vi "test_F9P_232-2.vi"() -> ()   [LabVIEW 2019]
panel:
  in  "cfg":T1={"Port"="COM5", "heading select"="NARROW_INT", "mode select"=["INS_RTKFIXED", "INS_RTKFLOAT"]}
  out "gps receive":string="$GNRMC,064134.00,A,3723.59859,N,12656.92614,E,0.021,,250720,,,A,V*12\r\n$GNVTG,,T,,M,0.021,N,0.039,K,A*34\r\n$GNGGA,064134.00,3723.59859,N,12656.92614,E,1,12,0.65,65.4,M,18.5,M,,*7E\r\n$GNGSA,A,3,17,19,06,05,02,12,09,,,,,,1.13,0.65,0.92,1*0F\r\n$GNGSA,A,3,85,70,71,72,,,,,,,,,1.13,0.65,0.92,2*00\r\n$GNGSA,A,3,36,19,11,04,09,12,,,,,,,1.13,0.65,0.92,3*0B\r\n$GNGSA,A,3,28,14,13,11,33,08,10,,,,,,1.13,0.65,0.92,4*0B\r\n$GPGSV,4,1,13,02,64,333,46,04,09,037,16,05,47,260,36,06,59,075,39,1*69\r\n$GPGSV,4,2,13,07,06,105,,09,39,058,39,12,18,264,15,13,07,191,,1*63\r\n$GPGSV,4,3,13,17,20,157,15,19,38,161,44,25,11,294,,29,06,323,,1*60\r\n$GPGSV,4,4,13,30,01,134,,1*52\r\n$GPGSV,4,1,13,02,64,333,,04,09,037,,05,47,260,36,06,59,075,37,6*65\r\n$GPGSV,4,2,13,07,06,105,,09,39,058,34,12,18,264,,13,07,191,,6*6D\r\n$GPGSV,4,3,13,17,20,157,,19,38,161,,25,11,294,,29,06,323,,6*63\r\n$GPGSV,4,4,13,30,01,134,,6*55\r\n$GLGSV,2,1,06,70,55,030,37,71,68,223,38,72,17,216,19,84,09,133,09,1*7E\r\n$GLGSV,2,2,06,85,64,109,38,86,50,337,,1*7E\r\n$GLGSV,2,1,06,70,55,030,,71,68,223,35,72,17,216,23,84,09,133,09,3*7C\r\n$GLGSV,2,2,06,85,64,109,33,86,50,337,,3*77\r\n$GAGSV,3,1,09,02,04,288,07,04,68,087,34,09,43,196,30,11,77,034,38,7*76\r\n$GAGSV,3,2,09,12,32,114,26,18,55,286,43,19,18,042,13,25,01,241,,7*7F\r\n$GAGSV,3,3,09,36,34,314,26,7*4A\r\n$GAGSV,3,1,09,02,04,288,,04,68,087,40,09,43,196,36,11,77,034,36,2*7F\r\n$GAGSV,3,2,09,12,32,114,16,18,55,286,46,19,18,042,,25,01,241,,2*7E\r\n$GAGSV,3,3,09,36,34,314,25,2*4C\r\n$GBGSV,4,1,13,04,35,133,,05,09,257,,06,27,182,,07,09,201,,1*7B\r\n$GBGSV,4,2,13,08,65,355,42,09,07,194,,10,16,222,,11,38,142,24,1*70\r\n$GBGSV,4,3,13,13,50,314,28,14,77,038,43,28,58,310,41,33,72,237,40,1*76\r\n$GBGSV,4,4,13,34,13,141,,1*45\r\n$GBGSV,4,1,13,04,35,133,,05,09,257,,06,27,182,,07,09,201,,3*79\r\n$GBGSV,4,2,13,08,65,355,43,09,07,194,,10,16,222,17,11,38,142,22,3*73\r\n$GBGSV,4,3,13,13,50,314,32,14,77,038,42,28,58,310,,33,72,237,,3*7F\r\n$GBGSV,4,4,13,34,13,141,,3*47\r\n$GNGLL,3723.59859,N,12656.92614,E,064134.00,A,A*70\r\n$GNRMC,064135.00,A,3723.59865,N,12656.92610,E,0.011,,250720,,,A,V*1B\r\n$GNVTG,,T,,M,0.011,N,0.020,K,A*3F\r\n$GNGGA,064135.00,3723.59865,N,12656.92610,E,1,12,0.65,65.2,M,18.5,M,,*72\r\n$GNGSA,A,3,17,19,06,05,02,12,09,,,,,,1.13,0.65,0.92,1*0F\r\n$GNGSA,A,3,85,70,71,72,,,,,,,,,1.13,0.65,0.92,2*00\r\n$GNGSA,A,3,36,19,11,04,09,12,,,,,,,1.13,0.65,0.92,3*0B\r\n$GNGSA,A,3,28,14,13,11,33,08,10,,,,,,1.13,0.65,0.92,4*0B\r\n$GPGSV,4,1,13,02,64,333,45,04,09,037,16,05,47,260,37,06,59,075,39,1*6B\r\n$GPGSV,4,2,13,07,06,105,,09,39,058,39,12,18,264,14,13,07,191,,1*62\r\n$GPGSV,4,3,13,17,20,157,16,19,38,161,44,25,11,294,,29,06,323,17,1*65\r\n$GPGSV,4,4,13,30,01,134,,1*52\r\n$GPGSV,4,1,13,02,64,333,,04,09,037,,05,47,260,35,06,59,075,37,6*66\r\n$GPGSV,4,2,13,07,06,105,,09,39,058,34,12,18,264,,13,07,191,,6*6D\r\n$GPGSV,4,3,13,17,20,157,,19,38,161,,25,11,294,,29,06,323,,6*63\r\n$GPGSV,4,4,13,30,01,134,,6*55\r\n$GLGSV,2,1,06,70,55,030,37,71,68,223,40,72,17,216,18,84,09,133,12,1*7A\r\n$GLGSV,2,2,06,85,64,109,38,86,50,337,,1*7E\r\n$GLGSV,2,1,06,70,55,030,,71,68,223,37,72,17,216,23,84,09,133,08,3*7F\r\n$GLGSV,2,2,06,85,64,109,33,86,50,337,,3*77\r\n$GAGSV,3,1,09,02,04,288,11,04,68,087,34,09,43,196,30,11,77,034,38,7*71\r\n$GAGSV,3,2,09,12,32,114,26,18,55,286,43,19,18,042,12,25,01,241,,7*7E\r\n$GAGSV,3,3,09,36,34,314,26,7*4A\r\n$GAGSV,3,1,09,02,04,288,,04,68,087,40,09,43,196,36,11,77,034,36,2*7F\r\n$GAGSV,3,2,09,12,32,114,16,18,55,286,47,19,18,042,,25,01,241,,2*7F\r\n$GAGSV,3,3,09,36,34,314,25,2*4C\r\n$GBGSV,4,1,13,04,35,133,,05,09,257,,06,27,182,,07,09,201,,1*7B\r\n$GBGSV,4,2,13,08,65,355,41,09,07,194,,10,16,222,,11,38,142,23,1*74\r\n$GBGSV,4,3,13,13,50,314,28,14,77,038,43,28,58,310,41,33,72,237,40,1*76\r\n$GBGSV,4,4,13,34,13,141,,1*45\r\n$GBGSV,4,1,13,04,35,133,,05,09,257,,06,27,182,,07,09,201,,3*79\r\n$GBGSV,4,2,13,08,65,355,43,09,07,194,,10,16,222,18,11,38,142,21,3*7F\r\n$GBGSV,4,3,13,13,50,314,31,14,77,038,41,28,58,310,,33,72,237,,3*7F\r\n$GBGSV,4,4,13,34,13,141,,3*47\r\n$GNGLL,3723.59865,N,12656.92610,E,064135.00,A,A*7A\r\n$GNRMC,064136.00,A,3723.59874,N,12656.92610,E,0.025,,250720,,,A,V*1F\r\n$GNVTG,,T,,M,0.025,N,0.046,K,A*38\r\n$GNGGA,064136.00,3723.59874,N,12656.92610,E,1,12,0.65,65.2,M,18.5,M,,*71\r\n$GNGSA,A,3,17,19,06,05,02,12,09,,,,,,1.13,0.65,0.92,1*0F\r\n$GNGSA,A,3,85,70,71,72,,,,,,,,,1.13,0.65,0.92,2*00\r\n$GNGSA,A,3,36,19,11,04,09,12,,,,,,,1.13,0.65,0.92,3*0B\r\n$GNGSA,A,3,28,14,13,11,33,08,10,,,,,,1.13,0.65,0.92,4*0B\r\n$GPGSV,4,1,13,02,64,333,43,04,09,037,15,05,47,260,30,06,59,075,36,1*66\r\n$GPGSV,4,2,13,07,06,105,,09,39,058,39,12,18,264,15,13,07,191,,1*63\r\n$GPGSV,4,3,13,17,20,157,14,19,38,161,41,25,11,294,,29,06,323,18,1*6D\r\n$GPGSV,4,4,13,30,01,134,,1*52\r\n$GPGSV,4,1,13,02,64,333,,04,09,037,,05,47,260,35,06,59,075,37,6*66\r\n$GPGSV,4,2,13,07,06,105,,09,39,058,34,12,18,264,,13,07,191,,6*6D\r\n$GPGSV,4,3,13,17,20,157,,19,38,161,,25,11,294,,29,06,323,,6*63\r\n$GPGSV,4,4,13,30,01,134,,6*55\r\n$GLGSV,2,1,06,70,55,030,35,71,68,223,38,72,17,216,17,84,09,133,09,1*72\r\n$GLGSV,2,2,06,85,64,109,34,86,50,337,,1*72\r\n$GLGSV,2,1,06,70,55,030,,71,68,223,37,72,17,216,24,84,09,133,11,3*70\r\n$GLGSV,2,2,06,85,64,109,35,86,50,337,,3*71\r\n$GAGSV,3,1,09,02,04,288,07,04,68,087,33,09,43,196,30,11,77,034,36,7*7F\r\n$GAGSV,3,2,09,12,32,114,26,18,55,286,41,19,18,042,13,25,01,241,,7*7D\r\n$GAGSV,3,3,09,36,34,314,27,7*4B\r\n$GAGSV,3,1,09,02,04,288,,04,68,087,40,09,43,196,37,11,77,034,36,2*7E\r\n$GAGSV,3,2,09,12,32,114,17,18,55,286,46,19,18,042,,25,01,241,,2*7F\r\n$GAGSV,3,3,09,36,34,314,25,2*4C\r\n$GBGSV,4,1,13,04,35,133,,05,09,257,,06,27,182,,07,09,201,,1*7B\r\n$GBGSV,4,2,13,08,65,355,40,09,07,194,,10,16,222,,11,38,142,22,1*74\r\n$GBGSV,4,3,13,13,50,314,28,14,77,038,41,28,58,310,42,33,72,237,39,1*79\r\n$GBGSV,4,4,13,34,13,141,,1*45\r\n$GBGSV,4,1,13,04,35,133,,05,09,257,,06,27,182,,07,09,201,,3*79\r\n$GBGSV,4,2,13,08,65,355,42,09,07,194,,10,16,222,19,11,38,142,19,3*74\r\n$GBGSV,4,3,13,13,50,314,31,14,77,038,41,28,58,310,,33,72,237,,3*7F\r\n$GBGSV,4,4,13,34,13,141,,3*47\r\n$GNGLL,3723.59874,N,12656.92610,E,064136.00,A,A*79\r\n$GNRMC,064137.00,A,3723.59883,N,12656.92607,E,0.046,,250720,,,A,V*15\r\n$GNVTG,,T,,M,0.046,N,0.085,K,A*32\r\n$GNGGA,064137.00,3723.59883,N,12656.92607,E,1,12,0.65,65.5,M,18.5,M,,*79\r\n$GNGSA,A,3,17,19,06,05,02,12,09,,,,,,1.13,0.65,0.92,1*0F\r\n$GNGSA,A,3,85,70,71,72,,,,,,,,,1.13,0.65,0.92,2*00\r\n$GNGSA,A,3,36,19,11,04,09,12,,,,,,,1.13,0.65,0.92,3*0B\r\n$GNGSA,A,3,28,14,13,11,33,08,10,,,,,,1.13,0.65,0.92,4*0B\r\n$GPGSV,4,1,13,02,64,333,46,04,09,037,12,05,47,260,32,06,59,075,43,1*64\r\n$GPGSV,4,2,13,07,06,105,,09,39,058,32,12,18,264,17,13,07,191,,1*6A\r\n$GPGSV,4,3,13,17,20,157,13,19,38,161,43,25,11,294,,29,06,323,17,1*67\r\n$GPGSV,4,4,13,30,01,134,,1*52\r\n$GPGSV,4,1,13,02,64,333,,04,09,037,,05,47,260,35,06,59,075,37,6*66\r\n$GPGSV,4,2,13,07,06,105,,09,39,058,35,12,18,264,,13,07,191,,6*6C\r\n$GPGSV,4,3,13,17,20,157,,19,38,161,,25,11,294,,29,06,323,,6*63\r\n$GPGSV,4,4,13,30,01,134,,6*55\r\n$GLGSV,2,1,06,70,55,030,36,71,68,223,42,72,17,216,18,84,09,133,09,1*73\r\n$GLGSV,2,2,06,85,64,109,37,86,50,337,,1*71\r\n$GLGSV,2,1,06,70,55,030,,71,68,223,36,72,17,216,24,84,09,133,10,3*70\r\n$GLGSV,2,2,06,85,64,109,33,86,50,337,,3*77\r\n$GAGSV,3,1,09,02,04,288,10,04,68,087,37,09,43,196,30,11,77,034,38,7*73\r\n$GAGSV,3,2,09,12,32,114,26,18,55,286,45,19,18,042,14,25,01,241,,7*7E\r\n$GAGSV,3,3,09,36,34,314,28,7*44\r\n$GAGSV,3,1,09,02,04,288,,04,68,087,40,09,43,196,37,11,77,034,37,2*7F\r\n$GAGSV,3,2,09,12,32,114,16,18,55,286,47,19,18,042,,25,01,241,,2*7F\r\n$GAGSV,3,3,09,36,34,314,25,2*4C\r\n$GBGSV,4,1,13,04,35,133,,05,09,257,,06,27,182,,07,09,201,,1*7B\r\n$GBGSV,4,2,13,08,65,355,40,09,07,194,,10,16,222,,11,38,142,21,1*77\r\n$GBGSV,4,3,13,13,50,314,29,14,77,038,43,28,58,310,41,33,72,237,40,1*77\r\n$GBGSV,4,4,13,34,13,141,,1*45\r\n$GBGSV,4,1,13,04,35,133,,05,09,257,,06,27,182,,07,09,201,,3*79\r\n$GBGSV,4,2,13,08,65,355,44,09,07,194,,10,16,222,18,11,38,142,18,3*72\r\n$GBGSV,4,3,13,13,50,314,32,14,77,038,42,28,58,310,,33,72,237,,3*7F\r\n$GBGSV,4,4,13,34,13,141,,3*47\r\n$GNGLL,3723.59883,N,12656.92607,E,064137.00,A,A*76\r\n$GNRMC,064138.00,A,3723.59888,N,12656.92600,E,0.018,,250720,,,A,V*1D\r\n$GNVTG,,T,,M,0.018,N,0.033,K,A*34\r\n$GNGGA,064138.00,3723.59888,N,12656.92600,E,1,12,0.70,65.3,M,18.5,M,,*78\r\n$GNGSA,A,3,17,19,06,05,02,09,,,,,,,1.20,0.70,0.98,1*02\r\n$GNGSA,A,3,85,70,71,72,,,,,,,,,1.20,0.70,0.98,2*0E\r\n$GNGSA,A,3,36,19,11,04,09,12,,,,,,,1.20,0.70,0.98,3*05\r\n$GNGSA,A,3,28,14,13,11,33,08,10,,,,,,1.20,0.70,0.98,4*05\r\n$GPGSV,4,1,13,02,64,333,45,04,09,037,,05,47,260,38,06,59,075,43,1*6E\r\n$GPGSV,4,2,13,07,06,105,,09,39,058,32,12,18,264,,13,07,191,,1*6C\r\n$GPGSV,4,3,13,17,20,157,15,19,38,161,42,25,11,294,,29,06,323,18,1*6F\r\n$GPGSV,4,4,13,30,01,134,,1*52\r\n$GPGSV,4,1,13,02,64,333,,04,09,037,,05,47,260,36,06,59,075,35,6*67\r\n$GPGSV,4,2,13,07,06,105,,09,39,058,34,12,18,264,,13,07,191,,6*6D\r\n$GPGSV,4,3,13,17,20,157,,19,38,161,,25,11,294,,29,06,323,,6*63\r\n$GPGSV,4,4,13,30,01,134,,6*55\r\n$GLGSV,2,1,06,70,55,030,40,71,68,223,42,72,17,216,19,84,09,133,14,1*7F\r\n$GLGSV,2,2,06,85,63,111,40,86,50,337,,1*7F\r\n$GLGSV,2,1,06,70,55,030,,71,68,223,36,72,17,216,25,84,09,133,09,3*79\r\n$GLGSV,2,2,06,85,63,111,28,86,50,337,,3*73\r\n$GAGSV,3,1,09,02,04,288,09,04,68,087,36,09,43,196,33,11,77,034,38,7*79\r\n$GAGSV,3,2,09,12,32,114,23,18,55,286,45,19,18,042,12,25,01,241,,7*7D\r\n$GAGSV,3,3,09,36,34,314,26,7*4A\r\n$GAGSV,3,1,09,02,04,288,,04,68,087,41,09,43,196,36,11,77,034,37,2*7F\r\n$GAGSV,3,2,09,12,32,114,15,18,55,286,48,19,18,042,,25,01,241,,2*73\r\n$GAGSV,3,3,09,36,34,314,24,2*4D\r\n$GBGSV,4,1,13,04,35,133,,05,09,257,,06,27,182,,07,09,201,,1*7B\r\n$GBGSV,4,2,13,08,65,355,40,09,07,194,,10,16,222,,11,38,142,21,1*77\r\n$GBGSV,4,3,13,13,50,314,32,14,77,038,43,28,58,310,43,33,72,237,41,1*7E\r\n$GBGSV,4,4,13,34,13,141,,1*45\r\n$GBGSV,4,1,13,04,35,133,,05,09,257,,06,27,182,,07,09,201,,3*79\r\n$GBGSV,4,2,13,08,65,355,44,09,07,194,,10,16,222,18,11,38,142,17,3*7D\r\n$GBGSV,4,3,13,13,50,314,31,14,77,038,43,28,58,310,,33,72,237,,3*7D\r\n$GBGSV,4,4,13,34,13,141,,3*47\r\n$GNGLL,3723.59888,N,12656.92600,E,064138.00,A,A*75\r\n$GNRMC,064139.00,A,3723.59894,N,12656.92597,E,0.040,,250720,,,A,V*11\r\n$GNVTG,,T,,M,0.040,N,0.073,K,A*3D\r\n$GNGGA,064139.00,3723.59894,N,12656.92597,E,1,12,0.76,65.2,M,18.5,M,,*7E\r\n$GNGSA,A,3,17,19,06,05,02,09,,,,,,,1.26,0.76,1.01,1*03\r\n$GNGSA,A,3,85,70,71,72,,,,,,,,,1.26,0.76,1.01,2*0F\r\n$GNGSA,A,3,36,19,11,04,09,12,,,,,,,1.26,0.76,1.01,3*04\r\n$GNGSA,A,3,28,14,13,11,33,08,10,,,,,,1.26,0.76,1.01,4*04\r\n$GPGSV,4,1,13,02,64,333,44,04,09,037,,05,47,260,37,06,59,075,40,1*63\r\n$GPGSV,4,2,13,07,06,105,,09,39,058,35,12,18,264,,13,07,191,,1*6B\r\n$GPGSV,4,3,13,17,20,157,14,19,38,161,42,25,11,294,,29,06,323,18,1*6E\r\n$GPGSV,4,4,13,30,01,134,,1*52\r\n$GPGSV,4,1,13,02,64,333,,04,09,037,,05,47,260,36,06,59,075,36,6*64\r\n$GPGSV,4,2,13,07,06,105,,09,39,058,37,12,18,264,,13,07,191,,6*6E\r\n$GPGSV,4,3,13,17,20,157,,19,38,161,,25,11,294,,29,06,323,,6*63\r\n$GPGSV,4,4,13,30,01,134,,6*55\r\n$GLGSV,2,1,06,70,55,030,39,71,68,223,43,72,17,216,21,84,09,133,11,1*7E\r\n$GLGSV,2,2,06,85,63,111,41,86,51,337,,1*7F\r\n$GLGSV,2,1,06,70,55,030,,71,68,223,35,72,17,216,24,84,09,133,08,3*7A\r\n$GLGSV,2,2,06,85,63,111,27,86,51,337,,3*7D\r\n$GAGSV,3,1,09,02,04,288,08,04,68,087,38,09,43,196,27,11,77,034,38,7*73\r\n$GAGSV,3,2,09,12,32,114,25,18,55,286,45,19,18,042,13,25,01,241,,7*7A\r\n$GAGSV,3,3,09,36,34,314,25,7*49\r\n$GAGSV,3,1,09,02,04,288,,04,68,087,41,09,43,196,37,11,77,034,37,2*7E\r\n$GAGSV,3,2,09,12,32,114,13,18,55,286,47,19,18,042,,25,01,241,,2*7A\r\n$GAGSV,3,3,09,36,34,314,24,2*4D\r\n$GBGSV,4,1,13,04,35,133,,05,09,257,,06,27,182,,07,09,201,,1*7B\r\n$GBGSV,4,2,13,08,65,355,39,09,07,194,,10,16,222,,11,38,142,20,1*78\r\n$GBGSV,4,3,13,13,50,314,33,14,77,038,42,28,58,310,40,33,72,237,41,1*7D\r\n$GBGSV,4,4,13,34,13,141,,1*45\r\n$GBGSV,4,1,13,04,35,133,,05,09,257,,06,27,182,,07,09,201,,3*79\r\n$GBGSV,4,2,13,08,65,355,44,09,07,194,,10,16,222,17,11,38,142,17,3*72\r\n$GBGSV,4,3,13,13,50,314,30,14,77,038,42,28,58,310,,33,72,237,,3*7D\r\n$GBGSV,4,4,13,34,13,141,,3*47\r\n$GNGLL,3723.59894,N,12656.92597,E,064139.00,A,A*74\r\n$GNRMC,064140.00,A,3723.59897,N,12656.92595,E,0.024,,250720,,,A,V*1C\r\n$GNVTG,,T,,M,0.024,N,0.044,K,A*3B\r\n$GNGGA,064140.00,3723.59897,N,12656.92595,E,1,12,0.76,64.8,M,18.5,M,,*7A\r\n$GNGSA,A,3,19,06,05,02,09,,,,,,,,1.26,0.76,1.01,1*05\r\n$GNGSA,A,3,85,70,71,72,,,,,,,,,1.26,0.76,1.01,2*0F\r\n$GNGSA,A,3,36,19,11,04,09,12,,,,,,,1.26,0.76,1.01,3*04\r\n$GNGSA,A,3,28,14,13,11,33,08,10,,,,,,1.26,0.76,1.01,4*04\r\n$GPGSV,4,1,13,02,64,333,47,04,09,037,,05,47,260,36,06,59,075,39,1*6F\r\n$GPGSV,4,2,13,07,06,105,,09,39,058,35,12,18,264,,13,07,191,,1*6B\r\n$GPGSV,4,3,13,17,20,157,,19,38,161,43,25,11,294,,29,06,323,18,1*6A\r\n$GPGSV,4,4,13,30,01,134,,1*52\r\n$GPGSV,4,1,13,02,64,333,,04,09,037,,05,47,260,36,06,59,075,34,6*66\r\n$GPGSV,4,2,13,07,06,105,,09,39,058,37,12,18,264,,13,07,191,,6*6E\r\n$GPGSV,4,3,13,17,20,157,,19,38,161,,25,11,294,,29,06,323,,6*63\r\n$GPGSV,4,4,13,30,01,134,,6*55\r\n$GLGSV,2,1,06,70,55,030,39,71,68,223,43,72,17,216,22,84,09,133,13,1*7F\r\n$GLGSV,2,2,06,85,63,111,42,86,51,337,,1*7C\r\n$GLGSV,2,1,06,70,55,030,,71,68,223,37,72,17,216,23,84,09,133,08,3*7F\r\n$GLGSV,2,2,06,85,63,111,28,86,51,337,,3*72\r\n$GAGSV,3,1,09,02,04,288,08,04,68,087,39,09,43,196,31,11,77,034,38,7*75\r\n$GAGSV,3,2,09,12,32,114,26,18,55,286,45,19,18,042,11,25,01,241,,7*7B\r\n$GAGSV,3,3,09,36,34,314,25,7*49\r\n$GAGSV,3,1,09,02,04,288,,04,68,087,38,09,43,196,37,11,77,034,37,2*70\r\n$GAGSV,3,2,09,12,32,114,12,18,55,286,47,19,18,042,,25,01,241,,2*7B\r\n$GAGSV,3,3,09,36,34,314,23,2*4A\r\n$GBGSV,4,1,13,04,35,133,,05,09,257,,06,27,182,,07,09,201,,1*7B\r\n$GBGSV,4,2,13,08,65,355,41,09,07,194,,10,16,222,,11,38,142,22,1*75\r\n$GBGSV,4,3,13,13,50,314,33,14,77,038,43,28,58,310,41,33,72,237,43,1*7F\r\n$GBGSV,4,4,13,34,13,141,,1*45\r\n$GBGSV,4,1,13,04,35,133,,05,09,257,,06,27,182,,07,09,201,,3*79\r\n$GBGSV,4,2,13,08,65,355,44,09,07,194,,10,16,222,16,11,38,142,17,3*73\r\n$GBGSV,4,3,13,13,50,314,31,14,77,038,41,28,58,310,,33,72,237,,3*7F\r\n$GBGSV,4,4,13,34,13,141,,3*47\r\n$GNGLL,3723.59897,N,12656.92595,E,064140.00,A,A*7B\r\n$GNRMC,064141.00,A,3723.59895,N,12656.92586,E,0.013,,250720,,,A,V*19\r\n$GNVTG,,T,,M,0.013,N,0.024,K,A*39\r\n$GNGGA,064141.00,3723.59895,N,12656.92586,E,1,12,0.76,64.6,M,18.5,M,,*75\r\n$GNGSA,A,3,19,06,05,02,09,,,,,,,,1.26,0.76,1.01,1*05\r\n$GNGSA,A,3,85,70,71,72,,,,,,,,,1.26,0.76,1.01,2*0F\r\n$GNGSA,A,3,36,19,11,04,09,12,,,,,,,1.26,0.76,1.01,3*04\r\n$GNGSA,A,3,28,14,13,11,33,08,10,,,,,,1.26,0.76,1.01,4*04\r\n$GPGSV,4,1,13,02,64,333,45,04,09,037,,05,47,260,39,06,59,075,42,1*6E\r\n$GPGSV,4,2,13,07,06,105,,09,39,058,,12,18,264,,13,07,191,,1*6D\r\n$GPGSV,4,3,13,17,20,157,18,19,38,161,42,25,11,294,,29,06,323,18,1*62\r\n$GPGSV,4,4,13,30,01,134,,1*52\r\n$GPGSV,4,1,13,02,64,333,,04,09,037,,05,47,260,36,06,59,075,34,6*66\r\n$GPGSV,4,2,13,07,06,105,,09,39,058,34,12,18,264,,13,07,191,,6*6D\r\n$GPGSV,4,3,13,17,20,157,,19,38,161,,25,11,294,,29,06,323,,6*63\r\n$GPGSV,4,4,13,30,01,134,,6*55\r\n$GLGSV,2,1,06,70,55,030,36,71,68,223,44,72,17,216,21,84,09,133,11,1*76\r\n$GLGSV,2,2,06,85,63,111,37,86,51,337,,1*7E\r\n$GLGSV,2,1,06,70,55,030,,71,68,223,37,72,17,216,23,84,09,133,10,3*76\r\n$GLGSV,2,2,06,85,63,111,33,86,51,337,,3*78\r\n$GAGSV,3,1,09,02,04,288,11,04,68,087,36,09,44,196,31,11,77,034,40,7*7A\r\n$GAGSV,3,2,09,12,32,114,26,18,55,286,46,19,18,042,09,25,01,241,,7*71\r\n$GAGSV,3,3,09,36,34,314,25,7*49\r\n$GAGSV,3,1,09,02,04,288,,04,68,087,40,09,44,196,37,11,77,034,36,2*79\r\n$GAGSV,3,2,09,12,32,114,11,18,55,286,47,19,18,042,,25,01,241,,2*78\r\n$GAGSV,3,3,09,36,34,314,22,2*4B\r\n$GBGSV,4,1,13,04,35,133,,05,09,257,,06,27,182,,07,09,201,,1*7B\r\n$GBGSV,4,2,13,08,65,355,41,09,07,194,,10,16,222,,11,38,142,22,1*75\r\n$GBGSV,4,3,13,13,50,314,30,14,77,038,43,28,58,310,42,33,72,237,42,1*7E\r\n$GBGSV,4,4,13,34,13,141,,1*45\r\n$GBGSV,4,1,13,04,35,133,,05,09,257,,06,27,182,,07,09,201,,3*79\r\n$GBGSV,4,2,13,08,65,355,44,09,07,194,,10,16,222,16,11,38,142,19,3*7D\r\n$GBGSV,4,3,13,13,50,314,31,14,77,038,41,28,58,310,,33,72,237,,3*7F\r\n$GBGSV,4,4,13,34,13,141,,3*47\r\n$GNGLL,3723.59895,N,12656.92586,E,064141.00,A,A*7A\r\n$GNRMC,064142.00,A,3723.59893,N,12656.92582,E,0.128,,250720,,,A,V*11\r\n$GNVTG,,T,,M,0.128,N,0.238,K,A*3F\r\n$GNGGA,064142.00,3723.59893,N,12656.92582,E,1,12,0.76,64.4,M,18.5,M,,*76\r\n$GNGSA,A,3,19,06,05,02,09,,,,,,,,1.26,0.76,1.01,1*05\r\n$GNGSA,A,3,85,70,71,72,,,,,,,,,1.26,0.76,1.01,2*0F\r\n$GNGSA,A,3,36,19,11,04,09,12,,,,,,,1.26,0.76,1.01,3*04\r\n$GNGSA,A,3,28,14,13,11,33,08,10,,,,,,1.26,0.76,1.01,4*04\r\n$GPGSV,4,1,13,02,64,333,46,04,09,037,,05,47,260,39,06,59,075,45,1*6A\r\n$GPGSV,4,2,13,07,06,105,,09,39,058,37,12,18,264,19,13,07,191,,1*61\r\n$GPGSV,4,3,13,17,20,157,21,19,38,161,42,25,11,294,,29,06,323,17,1*67\r\n$GPGSV,4,4,13,30,01,134,,1*52\r\n$GPGSV,4,1,13,02,64,333,,04,09,037,,05,47,260,35,06,59,075,36,6*67\r\n$GPGSV,4,2,13,07,06,105,,09,39,058,34,12,18,264,,13,07,191,,6*6D\r\n$GPGSV,4,3,13,17,20,157,,19,38,161,,25,11,294,,29,06,323,,6*63\r\n$GPGSV,4,4,13,30,01,134,,6*55\r\n$GLGSV,2,1,06,70,55,030,34,71,68,223,37,72,17,216,21,84,09,133,10,1*71\r\n$GLGSV,2,2,06,85,63,111,39,86,51,337,,1*70\r\n$GLGSV,2,1,06,70,55,030,,71,68,223,33,72,17,216,23,84,09,133,08,3*7B\r\n$GLGSV,2,2,06,85,63,111,36,86,51,337,,3*7D\r\n$GAGSV,3,1,09,02,04,288,08,04,68,087,33,09,44,196,27,11,77,034,39,7*7E\r\n$GAGSV,3,2,09,12,32,114,25,18,55,286,48,19,18,042,16,25,01,241,,7*72\r\n$GAGSV,3,3,09,36,34,314,24,7*48\r\n$GAGSV,3,1,09,02,04,288,,04,68,087,40,09,44,196,37,11,77,034,36,2*79\r\n$GAGSV,3,2,09,12,32,114,12,18,55,286,45,19,18,042,,25,01,241,,2*79\r\n$GAGSV,3,3,09,36,34,314,22,2*4B\r\n$GBGSV,4,1,13,04,35,133,,05,09,257,,06,27,182,,07,09,201,,1*7B\r\n$GBGSV,4,2,13,08,65,355,42,09,07,194,,10,16,222,,11,38,142,25,1*71\r\n$GBGSV,4,3,13,13,50,314,33,14,77,038,42,28,58,310,41,33,72,237,37,1*7D\r\n$GBGSV,4,4,13,34,13,141,,1*45\r\n$GBGSV,4,1,13,04,35,133,,05,09,257,,06,27,182,,07,09,201,,3*79\r\n$GBGSV,4,2,13,08,65,355,42,09,07,194,,10,16,222,16,11,38,142,20,3*71\r\n$GBGSV,4,3,13,13,50,314,30,14,77,038,41,28,58,310,,33,72,237,,3*7E\r\n$GBGSV,4,4,13,34,13,141,,3*47\r\n$GNGLL,3723.59893,N,12656.92582,E,064142.00,A,A*7B\r\n$GNRMC,064143.00,A,3723.59889,N,12656.92573,E,0.182,,250720,,,A,V*15\r\n$GNVTG,,T,,M,0.182,N,0.338,K,A*3E\r\n$GNGGA,064143.00,3723.59889,N,12656.92573,E,1,12,0.68,64.4,M,18.5,M,,*7D\r\n$GNGSA,A,3,17,19,06,05,02,09,,,,,,,1.17,0.68,0.95,1*02\r\n$GNGSA,A,3,85,70,71,72,,,,,,,,,1.17,0.68,0.95,2*0E\r\n$GNGSA,A,3,36,19,11,04,09,12,,,,,,,1.17,0.68,0.95,3*05\r\n$GNGSA,A,3,28,14,13,11,33,08,10,,,,,,1.17,0.68,0.95,4*05\r\n$GPGSV,4,1,13,02,64,333,44,04,09,037,,05,47,260,40,06,59,075,36,1*62\r\n$GPGSV,4,2,13,07,06,105,,09,39,058,33,12,18,264,19,13,07,191,,1*65\r\n$GPGSV,4,3,13,17,20,157,23,19,38,161,39,25,11,294,,29,06,323,16,1*68\r\n$GPGSV,4,4,13,30,01,134,,1*52\r\n$GPGSV,4,1,13,02,64,333,,04,09,037,,05,47,260,34,06,59,075,34,6*64\r\n$GPGSV,4,2,13,07,06,105,,09,39,058,33,12,18,264,,13,07,191,,6*6A\r\n$GPGSV,4,3,13,17,20,157,,19,38,161,,25,11,294,,29,06,323,,6*63\r\n$GPGSV,4,4,13,30,01,134,,6*55\r\n$GLGSV,2,1,06,70,55,030,33,71,68,223,25,72,17,216,22,84,09,133,10,1*76\r\n$GLGSV,2,2,06,85,63,111,30,86,51,337,,1*79\r\n$GLGSV,2,1,06,70,55,030,,71,68,223,35,72,17,216,24,84,09,133,11,3*72\r\n$GLGSV,2,2,06,85,63,111,33,86,51,337,,3*78\r\n$GAGSV,3,1,09,02,04,288,07,04,68,087,38,09,44,196,27,11,77,034,38,7*7B\r\n$GAGSV,3,2,09,12,32,114,23,18,55,286,44,19,18,042,14,25,01,241,,7*7A\r\n$GAGSV,3,3,09,36,34,314,25,7*49\r\n$GAGSV,3,1,09,02,04,288,,04,68,087,37,09,44,196,35,11,77,034,30,2*7D\r\n$GAGSV,3,2,09,12,32,114,13,18,55,286,45,19,18,042,,25,01,241,,2*78\r\n$GAGSV,3,3,09,36,34,314,23,2*4A\r\n$GBGSV,4,1,13,04,35,133,,05,09,257,,06,27,182,,07,09,201,,1*7B\r\n$GBGSV,4,2,13,08,65,355,40,09,07,194,,10,16,222,,11,38,142,25,1*73\r\n$GBGSV,4,3,13,13,50,314,29,14,77,038,42,28,58,310,
